vi "Configure.vi"(8 "error in (no error)":errorcluster, 9 "NI_ChannelName":string, 10 "Type":string) -> (0 "error out":errorcluster, 3 "APG out":refnum<class "APG.lvclass">)   [LabVIEW 2021, in "APG.lvclass"]
uses:
  APG.lvclass
  APG.lvclass/APG.ctl
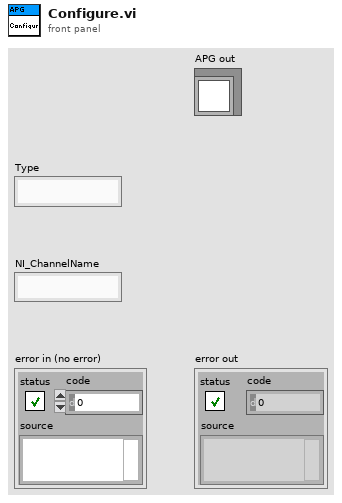
[diagram p1: front panel]
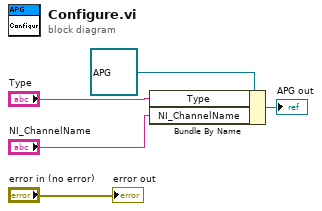
[diagram p0: block diagram]
diagram:
  n1 = Bundle By Name(cluster=refnum<class "APG.lvclass"> refnum ("APG in"), "Type"="Type", "NI_ChannelName"="NI_ChannelName") -> (→"APG out":refnum<class "APG.lvclass">)
  "error out" <- "error in (no error)"
